vi "String_Replace or Append.vi"(5 "Back(f)\nFront(t)":bool, 7 "Append(f)\nReplace(t)":bool, 10 "NewTest Data":string, 11 "Previeous String":string) -> (3 "New String Out":string)   [LabVIEW 2015]
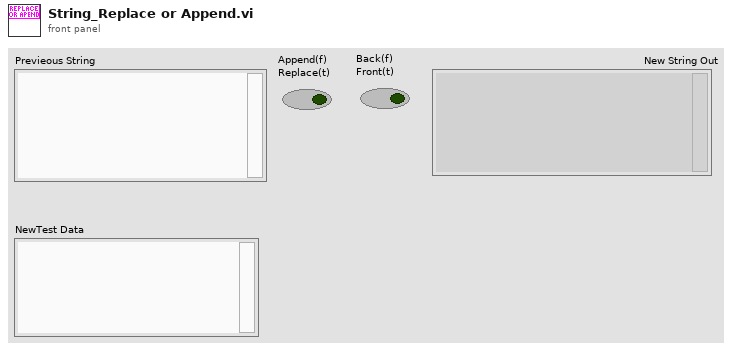
[diagram p1: front panel]
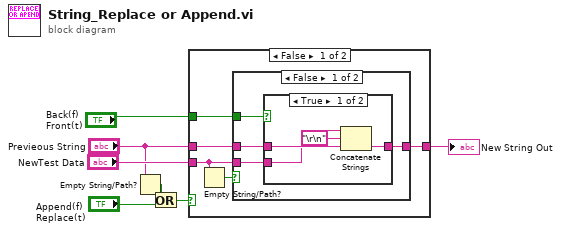
[diagram p0: block diagram]
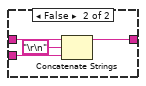
[diagram p2: hidden frame]
diagram:
  n1 = Empty String/Path?(string/path="Previeous String") -> (empty?=w3:bool)
  n2 = Or(x=w3, y="Append(f)\nReplace(t)") -> (x .or. y?=w2:bool)
  n3 = case shown="False" w2 {
    tunnel: "Previeous String" -> [w11 _]
    tunnel: [w12 w26] -> w5
    tunnel: "NewTest Data" -> [w10 w26]
    tunnel: "Back(f)\nFront(t)" -> [w8 _]
    frame False {
      n4 = Empty String/Path?(string/path=w10) -> (empty?=w9:bool)
      n5 = case shown="False" w9 {
        tunnel: [w16 w25] -> w12
        tunnel: w10 -> [w15 _]
        tunnel: w11 -> [w14 w25]
        tunnel: w8 -> [w13 _]
        frame False {
          n6 = case shown="True" w13 {
            tunnel: [w19 w24] -> w16
            tunnel: w15 -> [w17 w21]
            tunnel: w14 -> [w20 w22]
            frame True {
              n7 = Concatenate Strings(w17, "\r\n", w20) -> (w19:string)
            }
            frame False {
              n8 = Concatenate Strings(w22, "\r\n", w21) -> (w24:string)
            }
          }
        }
        frame True {
        }
      }
    }
    frame True {
    }
  }
  "New String Out" <- w5
